vi "Init Task.vi"(4 "counter":tag, 6 "line grouping":i32(ring) items=["one channel for each line", "one channel for all lines"], 7 "physical channels":tag, 8 "error in (no error)":errorcluster, 9 "name":string, 10 "DAQmxTaksContainer_General":refnum<class "DAQmxTaksContainer_General.lvclass">, 11 "DAQmxTaskDInput_Emulate in":refnum<class "DAQmxTaskDInput_Emulate.lvclass">) -> (0 "error out":errorcluster, 3 "DAQmxTaskDInput_Emulate OUT":refnum<class "DAQmxTaskDInput_Emulate.lvclass">)   [LabVIEW 2019, in "DAQmxTaskDInput_Emulate.lvclass"]
uses:
  DAQmxTaskDInput_Emulate.lvclass
  C:/Users/elysium/Documents/dev/TRANCON/Classes/DAQmxTasks/DAQmxTask.lvclass
  DAQmxTaskContainer_General/DAQmxTaksContainer_General.lvclass
  DAQmxTask.lvclass/DAQmxTask.ctl
  DAQmxTask.lvclass
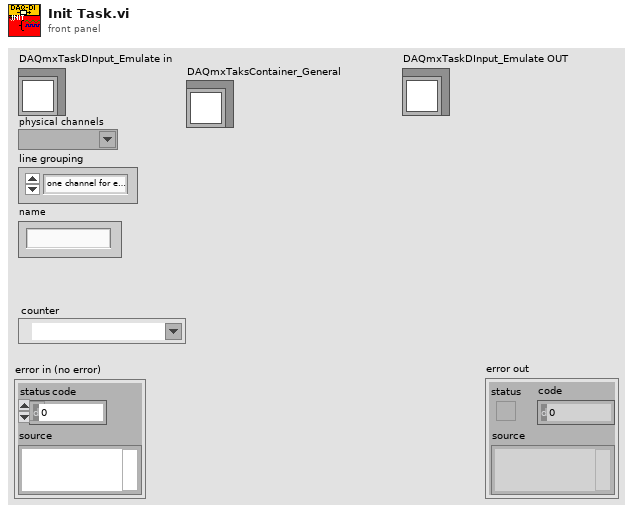
[diagram p1: front panel]
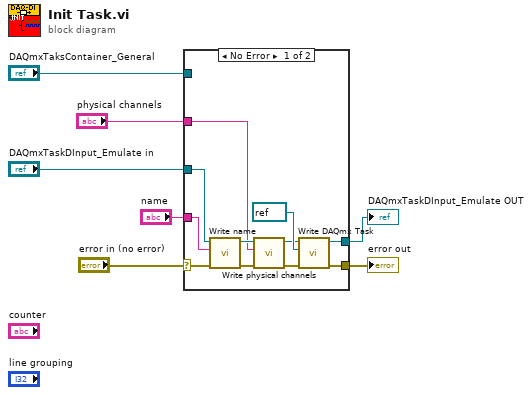
[diagram p0: block diagram]
diagram:
  n1 = case shown="No Error" "error in (no error)" {
    selector: "error in (no error)" -> [w13 w20]
    tunnel: "name" -> [w10 _]
    tunnel: "DAQmxTaskDInput_Emulate in" -> [w12 w19]
    tunnel: [w8 w20] -> w4
    tunnel: "physical channels" -> [w11 _]
    tunnel: "DAQmxTaksContainer_General" -> [_ _]
    tunnel: [w9 w19] -> w1
    frame No Error {
      n2 = call "Write name.vi"("error in (no error)"=w13, "name"=w10, "DAQmxTask in"=w12) -> ("error out"=w15:errorcluster, "DAQmxTask out"=w16:refnum<class "DAQmxTaskDInput_Emulate.lvclass">)  [unwired: 7 in]
      n3 = call "Write physical channels.vi"("error in (no error)"=w15, "physical channels"=w11, "DAQmxTask in"=w16) -> ("error out"=w14:errorcluster, "DAQmxTask out"=w17:refnum<class "DAQmxTaskDInput_Emulate.lvclass">)  [unwired: 7 in]
      n4 = call "Write DAQmx Task.vi"("error in (no error)"=w14, "DAQmx Task Name"=refnum<k21> refnum, "DAQmxTask in"=w17) -> ("error out"=w8:errorcluster, "DAQmxTask out"=w9:refnum<class "DAQmxTaskDInput_Emulate.lvclass">)  [unwired: 7 in]
    }
    frame Error {
    }
  }
  "error out" <- w4
  "DAQmxTaskDInput_Emulate OUT" <- w1
